vi "总氮断电保存全局变量.vi"() -> ()   [LabVIEW 2016, in "总氮.lvlib"]
panel:
  in  "质控参数设置":T1
  in  "总氮自动测试量程配置":T2={"水样测试量程模式"=enum."AUTO", "空白核查量程模式"=enum."AUTO", "跨度核查量程模式"=enum."AUTO"}
  out "曲线模型":T3={"XY图"=[], "标液浓度1"=0.0, "测量吸光度1"=0.0, "测量吸光度2"=0.0, "标液浓度2"=0.0, "测量吸光度3"=0.0, "标液浓度3"=0.0, "测量吸光度4"=0.0, "标液浓度4"=0.0, "测量吸光度5"=0.0, "标液浓度5"=0.0, "样品1启用"=FALSE, "样品3启用"=FALSE, "样品4启用"=FALSE, "样品5启用"=FALSE, "样品2启用"=FALSE, "拟合公式"="", "r^2"=0.0, "模型"=enum."线性", "method"=0, "样品1 F0"=0.0, "样品1 F1"=0.0, "样品2 F1"=0.0, "样品2 F0"=0.0, "样品3 F1"=0.0, "样品3 F0"=0.0, "样品4 F0"=0.0, "样品4 F1"=0.0, "样品5 F1"=0.0, "样品5 F0"=0.0, "精度"=4.0} {"method" items=["最小二乘", "最小绝对残差", "Bisquare"]; "r^2" format="%.7g"}
  in  "定时控制":T4
  # "质控参数设置"
  # "监测参数"
  # "总氮"
  # "跨度值"
  # "零点核查标准液浓度"
  # "跨度核查标准液浓度"
  # "标样核查标准液浓度"
  # "标液浓度"
  # "F0"
  # "F1"
  # "吸光值显示"
  # "样品一"
  # "辅\n助\n计\n算\n区"
  # "样品二"
  # "样品三"
  # "样品四"
  # "样品五"
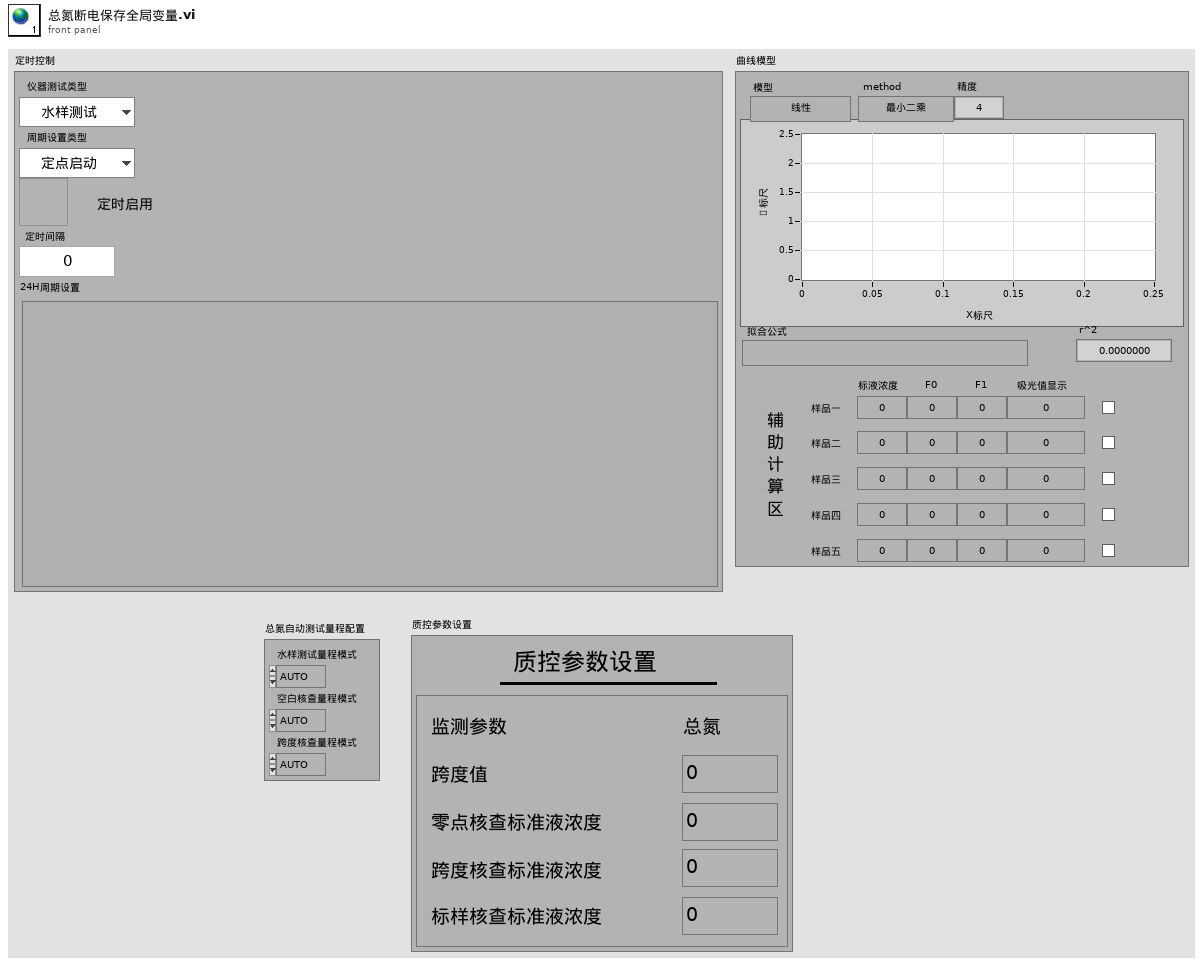
[diagram p1: front panel]
types:
  T1 = cluster{"跨度值":dbl, "零点标准液浓度":dbl, "跨度标准液浓度":dbl, "标准液标准浓度":dbl}
  T2 = cluster{"水样测试量程模式":enum16{"H", "L", "AUTO"}, "空白核查量程模式":enum16{"H", "L", "AUTO"}, "跨度核查量程模式":enum16{"H", "L", "AUTO"}}
  T3 = cluster{"XY图":cluster{"X Values":dbl[], "Y Values":dbl[]}[], "标液浓度1":dbl, "测量吸光度1":dbl, "测量吸光度2":dbl, "标液浓度2":dbl, "测量吸光度3":dbl, "标液浓度3":dbl, "测量吸光度4":dbl, "标液浓度4":dbl, "测量吸光度5":dbl, "标液浓度5":dbl, "样品1启用":bool, "样品3启用":bool, "样品4启用":bool, "样品5启用":bool, "样品2启用":bool, "拟合公式":string, "r^2":dbl, "模型":enum32{"线性", "多项式"}, "method":u16, "样品1 F0":dbl, "样品1 F1":dbl, "样品2 F1":dbl, "样品2 F0":dbl, "样品3 F1":dbl, "样品3 F0":dbl, "样品4 F0":dbl, "样品4 F1":dbl, "样品5 F1":dbl, "样品5 F0":dbl, "精度":dbl}
  T4 = cluster{"仪器测试类型":enum16{"水样测试", "标样核查", "空白测试", "跨度核查"}, "周期设置类型":enum16{"定点启动", "间隔启动"}, "定时功能启用":bool, "定时间隔":dbl, "24H周期设置":bool[]}
diagram:
